vi "mmW ZMQ Handle incomming messages.vi"(11 "module loopdata":T1) -> (0 "error out":errorcluster, 3 "OK":bool)   [LabVIEW 2019, in "Communication Interface.lvlib"]
doc: "ZMQ REP:\nRecieves messages from API as ZMQ REP Socket\nParses message content into commands and triggers command user event\nWaits for command response and forwards that response back to API\nvia ZMQ"
uses:
  Communication Interface.lvlib
  module data.ctl
  Intertarget communication/CR_master_class/CR_master.lvclass
  Intertarget communication/CR slave_class/CR slave.lvclass
  ZMQ_mmWave_class/ZMQ_mmWave.lvclass
  C:/Barkhausen mmWave radar/Development/modules/mmw_instrument/src_LabVIEW/Host/Intertarget communication/CR slave_class/CR slave.lvclass
  mmw_command_lib/src_LabVIEW/mmW_commands/TypeDefs/commands.ctl
  mmw_command_lib/src_LabVIEW/mmW_commands/replies/reply_statuscode.ctl
  Intertarget communication/Error response.ctl
  mmw_command_lib/src_LabVIEW/mmW_commands/commands/typedefs/mode.ctl
  SubVIs/Shared/CMD Configure RF.ctl
  SubVIs/Shared/CMD SetFS.ctl
  SubVIs/Shared/CMD Enable.ctl
  <vilib>/event_ctls.llb/usereventprio.ctl
  SubVIs/Shared/CMD Start.ctl
  mmw_command_lib/src_LabVIEW/mmW_commands/commands/typedefs/datatypes_.ctl
  SubVIs/Shared/CMD Trigger burst.ctl
  SubVIs/mmWave instrument_class/BurstMode.ctl
  SubVIs/IQBurst_memo_class/IQBurst_memo.lvclass
  C:/Barkhausen mmWave radar/Development/modules/mmw_instrument/src_LabVIEW/Host/SubVIs/mmWave data_class/mmWave data.lvclass
  mmw_command_lib/src_LabVIEW/mmW_commands/commands/typedefs/burst_mode.ctl
  mmw_command_lib/src_LabVIEW/mmW_commands/TypeDefs/response status.ctl
  SubVIs/Shared/Config state.ctl
  SubVIs/mmWave instrument_class/System info.ctl
  SubVIs/mmWave instrument_class/System state.ctl
  SubVIs/mmWave instrument_class/Instrument state.ctl
  SubVIs/mmWave instrument_class/Instrument mode.ctl
  SubVIs/mmWave instrument_class/Sync mode.ctl
  SubVIs/mmWave instrument_class/RF port info.ctl
  4d978cd8-de24-491d-9e02-cf2f9c928746.vi
  97d28283-8354-4fd1-aa63-0fed811ffe26.vi
  <vilib>/Utility/High Resolution Relative Seconds.vi
  <vilib>/Utility/error.llb/Clear Errors.vi
  SubVIs/Shared/Comm GV.vi
  SubVIs/Shared/System GV.vi
  Log/Log GV.vi
  SubVIs/Shared/Shared.lvlib
  mmw_command_lib/src_LabVIEW/mmW_commands/mmW_commands.lvlib
  <vilib>/addons/_JKI.lib/Serialization/JSON/JKI JSON Serialization.lvlib
  SubVIs/mmWave instrument_class/mmWave instrument.lvclass
  Intertarget communication/CommandResponse communication.lvlib
  Log/Log.lvlib
panel:
  out "fs (Hz)":dbl=3072000000.0
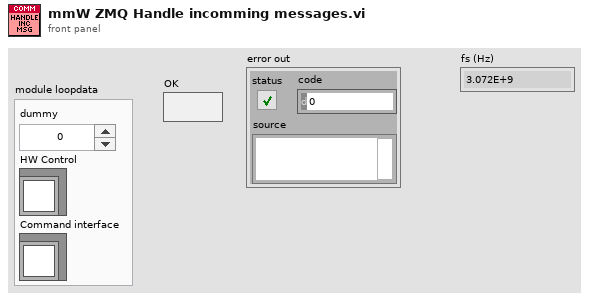
[diagram p1: front panel]
types:
  T1 = typedef "Communication Interface.lvlib/module data.ctl" = cluster{"dummy":dbl, "HW Control":refnum<class "CR_master.lvclass">, "Command interface":refnum<class "CR slave.lvclass">}
  T2 = typedef "mmW_commands.lvlib/commands.ctl" = enum16{"configure_fs", "configure_rf", "configure_trigger", "equalization_enable", "equalization_start", "lo_sync_enable", "equalization_stop", "get_instrument_status", "get_versions", "initialize_hw", "pop_rx", "set_log_level", "Shutdown", "start", "start_instrument_app", "stop", "trans", "transceive", "trigger_burst", "trigger_sync_enable", "Write TX", "resp_generic", "resp_waveform", "send_trigger", "fetch", "transceive2"}
  T3 = typedef "mmW_commands.lvlib/reply_statuscode.ctl" = enum16{"Error", "OK"}
  T4 = typedef "mmW_commands.lvlib/datatypes_.ctl" = enum16{"none", "string", "interleaved_I16", "interleaved_I32", "I16_array", "I32_array", "JSONstring"}
  T5 = typedef "mmW_commands.lvlib/response status.ctl" = enum16{"OK", "Error", "Warning", "Unknown"}
  T6 = typedef "CommandResponse communication.lvlib/Error response.ctl" = cluster{"code":i32, "message":string, "source":string}
  T7 = typedef "mmW_commands.lvlib/mode.ctl" = enum16{"RF", "IF", "BB"}
  T8 = typedef "Shared.lvlib/CMD Configure RF.ctl" = cluster{"port":string, "fc":dbl, "gain":dbl}
  T9 = typedef "Shared.lvlib/CMD SetFS.ctl" = cluster{"port":string, "fs":dbl}
  T10 = typedef "Shared.lvlib/CMD Enable.ctl" = cluster{"Enable":bool}
  T11 = typedef "usereventprio.ctl" = enum32{"high priority", "normal priority"}
  T12 = typedef "Shared.lvlib/CMD Start.ctl" = cluster{"Bursts":string[], "Acquisition duration":dbl}
  T13 = typedef "Shared.lvlib/CMD Trigger burst.ctl" = cluster{"Burst name":string, "Burst mode":T14}
  T14 = typedef "mmWave instrument.lvclass/BurstMode.ctl" = enum16{"burst", "continuous"}
  T15 = typedef "mmW_commands.lvlib/ports.ctl" = enum16{"rx", "tx"}
  T16 = cluster{"Boolean Round":bool, "code":i32, "source":string}
  T17 = typedef "mmW_commands.lvlib/burst_mode.ctl" = enum16{"burst", "continuous"}
  T18 = typedef "Shared.lvlib/Config state.ctl" = cluster{"system info":T19, "state":T20, "tx":T24, "rx":T24, "versions":cluster{"app":string, "tx fpga":string, "rx fpga":string}}
  T19 = typedef "mmWave instrument.lvclass/System info.ctl" = cluster{"mmw instr":string, "max fs":dbl, "RX/LO1 src":string, "TX/LO1 src":string, "LO2 src":string, "RX LO1 export":bool, "TX LO1 export":bool, "LO2 export":bool, "TX LO1 export level":dbl, "RX LO1 export level":dbl, "LO2 export level":dbl}
  T20 = typedef "mmWave instrument.lvclass/System state.ctl" = cluster{"hw state":T21, "lo sync en":bool, "trig sync en":bool, "mode":T22, "sync":T23, "equalization en":bool}
  T21 = typedef "mmWave instrument.lvclass/Instrument state.ctl" = enum16{"Off", "Initialization", "Configuration", "Running", "Calibration"}
  T22 = typedef "mmWave instrument.lvclass/Instrument mode.ctl" = enum16{"RF", "IF", "BB"}
  T23 = typedef "mmWave instrument.lvclass/Sync mode.ctl" = enum16{"Slave", "Master"}
  T24 = typedef "mmWave instrument.lvclass/RF port info.ctl" = cluster{"fc":dbl, "gain":dbl, "fs":dbl, "trigger delay":dbl}
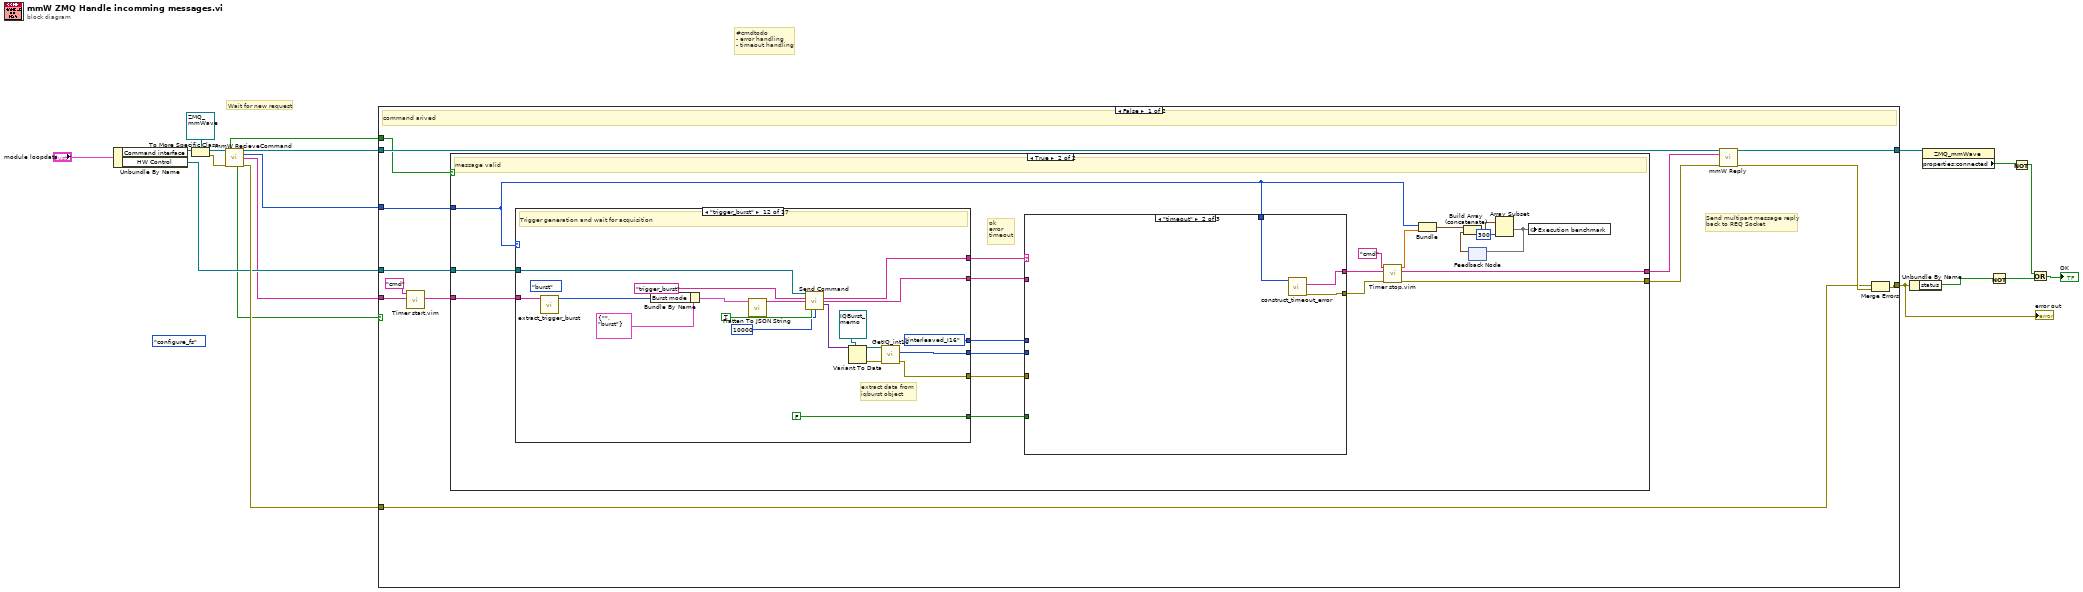
[diagram p0: block diagram]
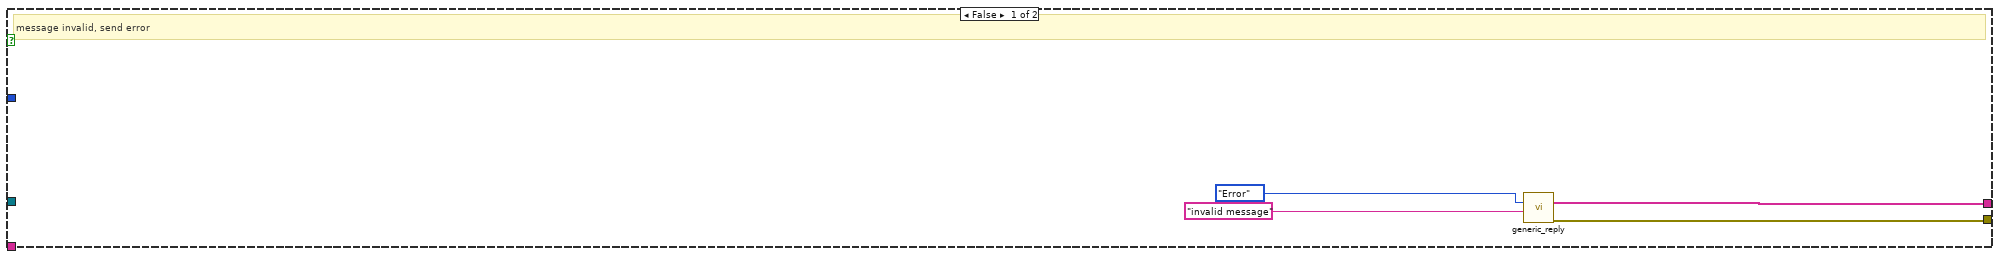
[diagram p2: hidden frame]
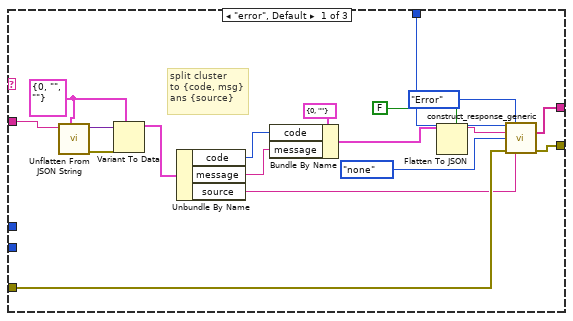
[diagram p3: hidden frame]
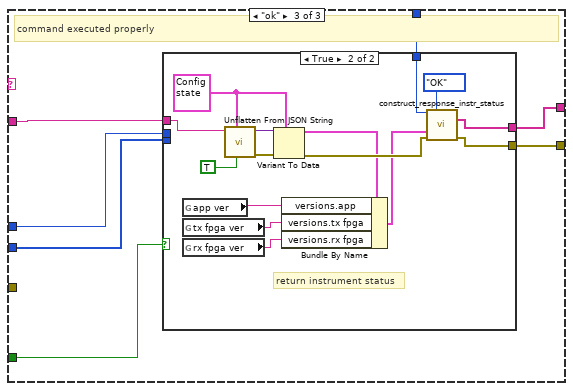
[diagram p4: hidden frame]
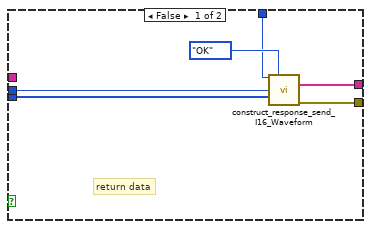
[diagram p5: hidden frame]
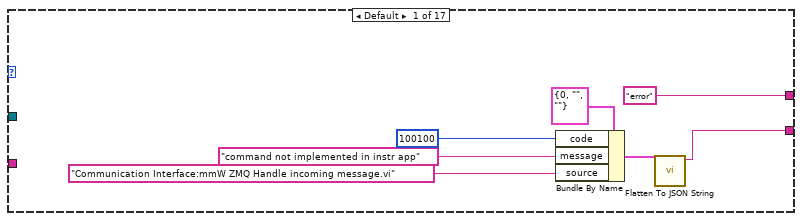
[diagram p6: hidden frame]
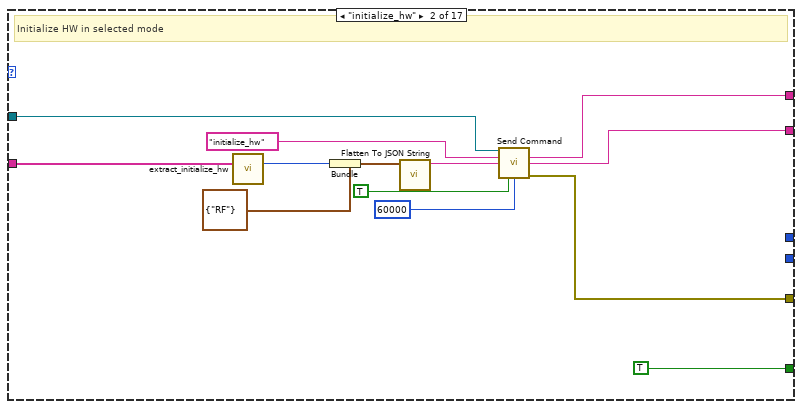
[diagram p7: hidden frame]
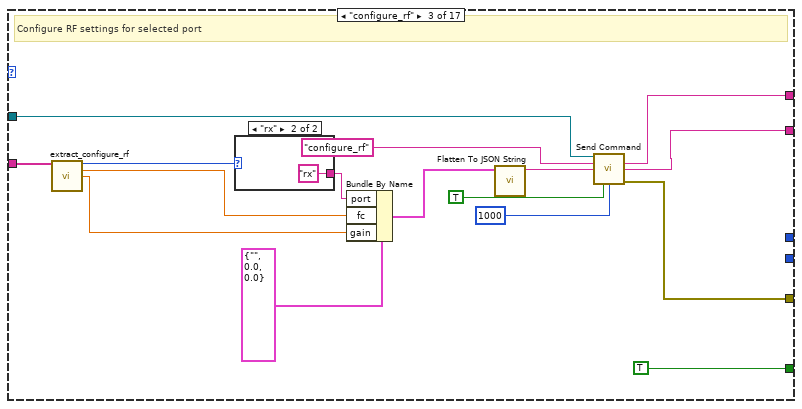
[diagram p8: hidden frame]
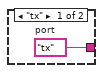
[diagram p9: hidden frame]
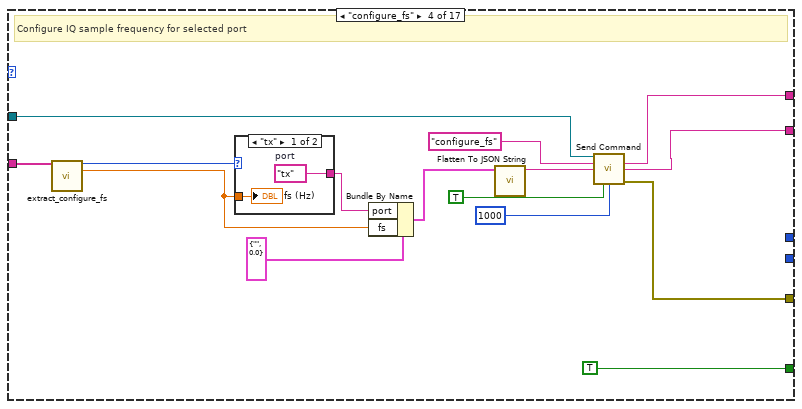
[diagram p10: hidden frame]
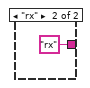
[diagram p11: hidden frame]
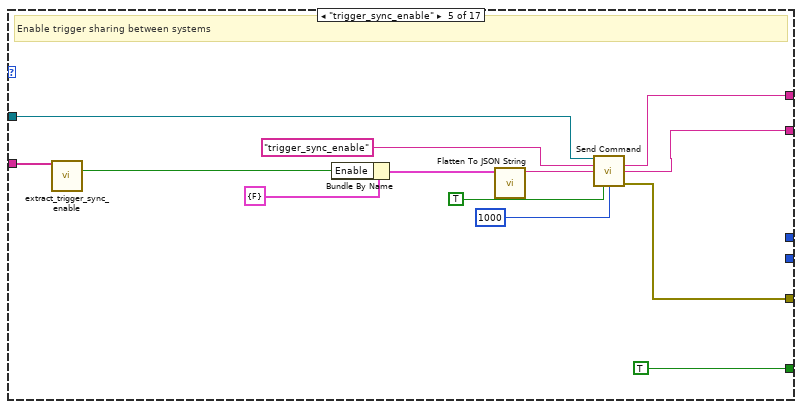
[diagram p12: hidden frame]
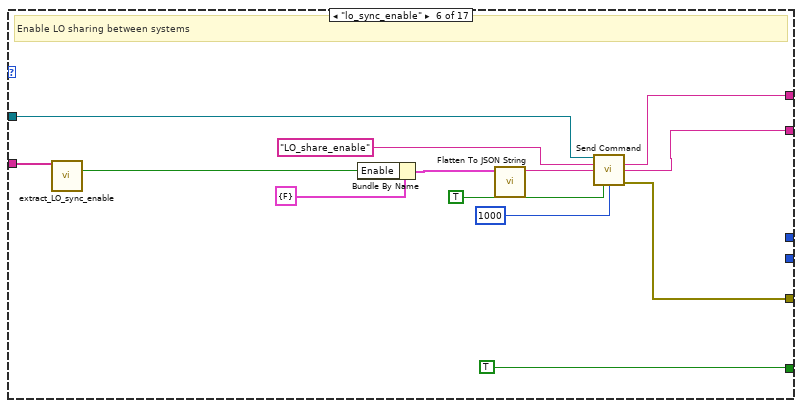
[diagram p13: hidden frame]
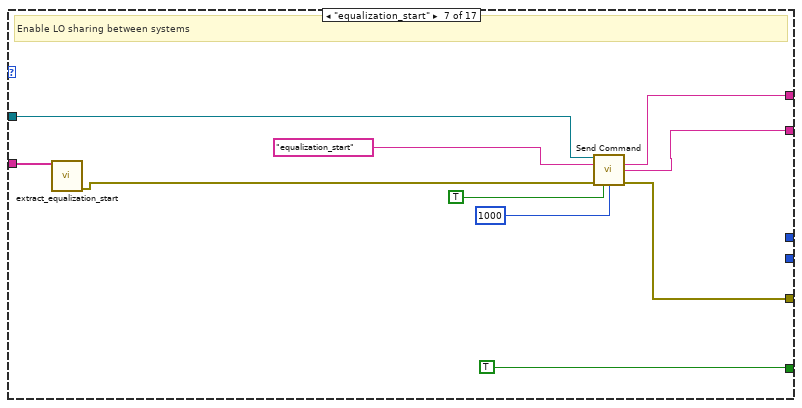
[diagram p14: hidden frame]
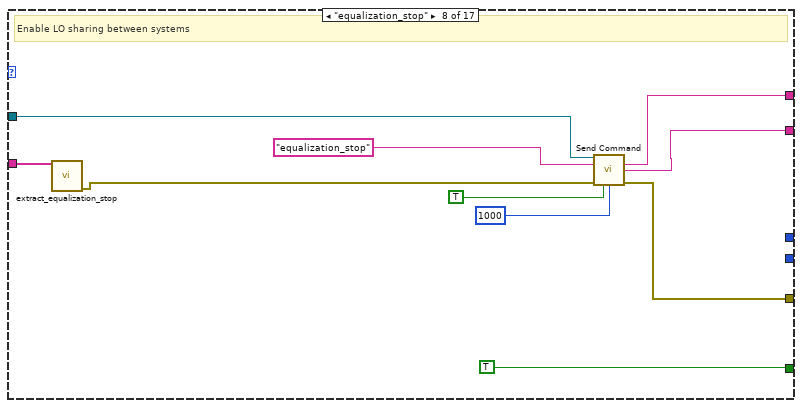
[diagram p15: hidden frame]
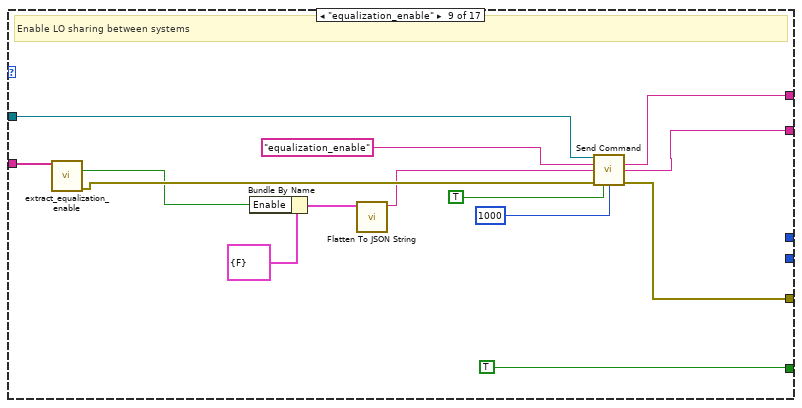
[diagram p16: hidden frame]
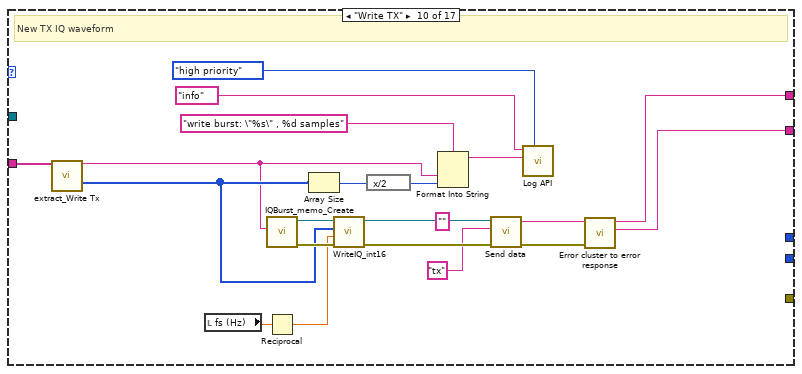
[diagram p17: hidden frame]
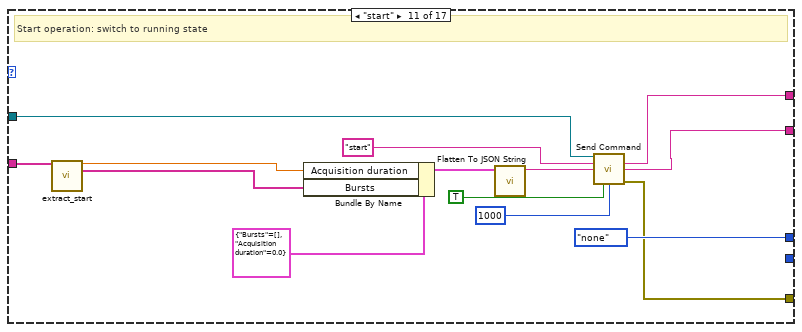
[diagram p18: hidden frame]
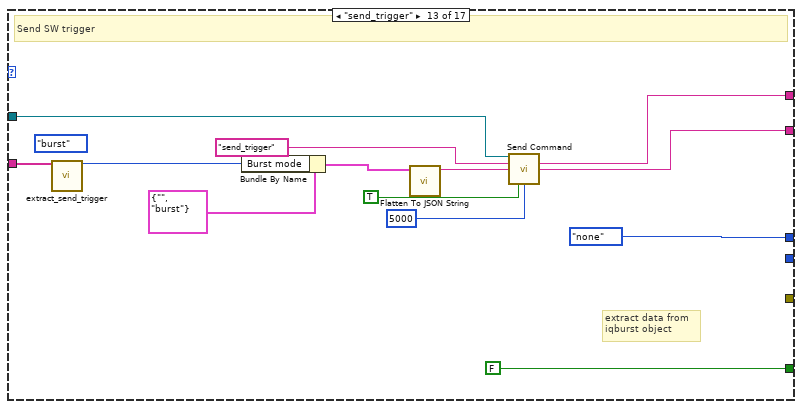
[diagram p19: hidden frame]
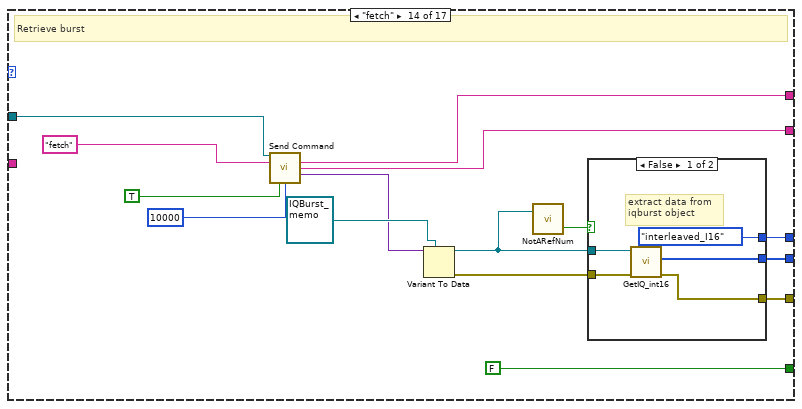
[diagram p20: hidden frame]
diagram:
  (unwired) commands."configure_fs" ("command out")
  # "Wait for new request"
  # "#cmdtodo\n- error handling\n- timeout handling"
  n1 = Unbundle By Name("module loopdata") -> ("Command interface"=w10:refnum<class "CR slave.lvclass">, "HW Control"=w11:refnum<class "CR_master.lvclass">)
  n2 = To More Specific Class(target class=refnum<class "ZMQ_mmWave.lvclass"> refnum ("CommandResponse communication.lvlib:ZMQ_mmWave"), reference=w10) -> (specific class reference=w8:refnum<class "ZMQ_mmWave.lvclass">, error out=w3:errorcluster)  [unwired: 1 in]
  n3 = call-dynamic "mmW RecieveCommand.vi"("reference in"=w8, "error in (no error)"=w3) -> ("Valid message?"=w2:bool, "reference out"=w12:refnum<class "ZMQ_mmWave.lvclass">, "command out"=w5:T2, "multipart message"=w4:string[], "timed out?"=w6:bool, "error out"=w13:errorcluster)  [unwired: 8 in]
  n4 = case shown="False" w6 {
    tunnel: w11 -> [w32 _]
    tunnel: w12 -> [w31 w359]
    tunnel: w13 -> [w27 w360]
    tunnel: [w28 w360] -> w14
    tunnel: [w30 w359] -> w15
    tunnel: w5 -> [w26 _]
    tunnel: w4 -> [w22 _]
    tunnel: w2 -> [w25 _]
    frame False {
      # "Send multipart message reply\nback to REQ Socket"
      # "command arived"
      n5 = call "Timer start.vim"("dataflow in"=w22, "timer in (t1)"="cmd" ("timer name (t1)")) -> ("dataflow out"=w21:string[])  [unwired: 8 in, 1 out]
      n6 = case shown="True" w25 {
        tunnel: w32 -> [_ w55]
        tunnel: w26 -> [_ w44]
        tunnel: w21 -> [_ w54]
        tunnel: [w36 w45] -> w24
        tunnel: [w33 w50] -> w23
        frame False {
          # "message invalid, send error"
          n7 = call "generic_reply.vi"("Status (Error)"=reply_statuscode."Error", "(error code)"="invalid message" ("Response out")) -> ("multipart message"=w36:string[], "error out"=w33:errorcluster)  [unwired: 11 in, 1 out]
        }
        frame True {
          # "ok\nerror\ntimeout"
          # "message valid"
          n8 = case shown="\"trigger_burst\"" w44 {
            tunnel: w55 -> [_ w114 w135 w152 w168 w181 w192 w202 w216 _ w249 w268 w281 w287 w313 w348 _]
            tunnel: w54 -> [_ w122 w140 w157 w173 w186 w196 w206 w220 w231 w254 w273 w286 _ w317 w347 _]
            tunnel: ["error" ("status") w116 w129 w147 w166 w179 w191 w201 w215 w234 w246 w255 w274 w288 w310 w346 _] -> w53
            tunnel: [w105 w115 w128 w146 w165 w178 w190 w200 w214 w233 w245 w265 w278 w298 w312 w345 _] -> w52
            tunnel: [_ _ _ _ _ _ _ _ _ _ _ w259 _ w294 _ w343 _] -> w51
            tunnel: [_ _ _ _ _ _ _ _ _ _ datatypes_."none" ("datatype") datatypes_."interleaved_I16" ("datatype") datatypes_."none" ("datatype") w293 _ w344 _] -> w49
            tunnel: [_ w113 w126 w145 w164 w177 w189 w199 w213 _ w241 w257 _ w292 w311 w326 _] -> w48
            tunnel: [_ TRUE TRUE TRUE TRUE TRUE TRUE TRUE TRUE _ _ FALSE FALSE FALSE _ _ _] -> w42
            frame Default {
              n9 = Bundle By Name(cluster=T6 {"code"=0, "message"="", "source"=""} ("Error response"), "code"=100100, "message"="command not implemented in instr app", "source"="Communication Interface:mmW ZMQ Handle incoming message.vi" ("message")) -> (w106:T6)
              n10 = call <vilib>:"Flatten To JSON String.vi"("Variant"=w106) -> ("JSON String"=w105:string)  [unwired: 9 in, 1 out]
            }
            frame "initialize_hw" {
              # "Initialize HW in selected mode"
              n11 = call "extract_initialize_hw.vi"("multipart message in"=w122) -> ("Mode"=w120:T7)  [unwired: 10 in, 4 out]
              n12 = Bundle(cluster=cluster{"mode":T7} {"mode"=enum."RF"}, "mode"=w120) -> (w118:cluster{"mode":T7})
              n13 = call <vilib>:"Flatten To JSON String.vi"("Variant"=w118) -> ("JSON String"=w119:string)  [unwired: 9 in, 1 out]
              n14 = call-dynamic "Send Command.vi"("reference in"=w114, "message"="initialize_hw", "parameters"=w119, "response?"=TRUE, "timeout"=60000) -> ("status"=w116:string, "reponse"=w115:string, "error out"=w113:errorcluster)  [unwired: 6 in, 2 out]
            }
            frame "configure_rf" {
              # "Configure RF settings for selected port"
              n15 = call "extract_configure_rf.vi"("multipart message in"=w140) -> ("ports"=w133:T15, "fc (Hz)"=w132:dbl, "gain"=w127:dbl)  [unwired: 9 in, 3 out]
              n16 = case shown="\"rx\"" w133 {
                tunnel: [w141 "rx" ("port")] -> w131
                frame "tx" {
                  w141 = "tx"  # port
                }
                frame "rx" {
                }
              }
              n17 = Bundle By Name(cluster=T8 {"port"="", "fc"=0.0, "gain"=0.0}, "port"=w131, "fc"=w132, "gain"=w127) -> (w130:T8)
              n18 = call <vilib>:"Flatten To JSON String.vi"("Variant"=w130) -> ("JSON String"=w136:string)  [unwired: 9 in, 1 out]
              n19 = call-dynamic "Send Command.vi"("reference in"=w135, "message"="configure_rf", "parameters"=w136, "response?"=TRUE, "timeout"=1000) -> ("status"=w129:string, "reponse"=w128:string, "error out"=w126:errorcluster)  [unwired: 6 in, 2 out]
            }
            frame "configure_fs" {
              # "Configure IQ sample frequency for selected port"
              n20 = call "extract_configure_fs.vi"("multipart message in"=w157) -> ("ports"=w150:T15, "fs (Hz)"=w143:dbl)  [unwired: 10 in, 3 out]
              n21 = case shown="\"tx\"" w150 {
                tunnel: [w159 "rx" ("port")] -> w149
                tunnel: w143 -> [w158 _]
                frame "tx" {
                  w159 = "tx"  # port
                  "fs (Hz)" <- w158
                }
                frame "rx" {
                }
              }
              n22 = Bundle By Name(cluster=T9 {"port"="", "fs"=0.0}, "port"=w149, "fs"=w143) -> (w148:T9)
              n23 = call <vilib>:"Flatten To JSON String.vi"("Variant"=w148) -> ("JSON String"=w153:string)  [unwired: 9 in, 1 out]
              n24 = call-dynamic "Send Command.vi"("reference in"=w152, "message"="configure_fs", "parameters"=w153, "response?"=TRUE, "timeout"=1000) -> ("status"=w147:string, "reponse"=w146:string, "error out"=w145:errorcluster)  [unwired: 6 in, 2 out]
            }
            frame "trigger_sync_enable" {
              # "Enable trigger sharing between systems"
              n25 = call "extract_trigger_sync_enable.vi"("multipart message in"=w173) -> ("Enable"=w162:bool)  [unwired: 11 in, 3 out]
              n26 = Bundle By Name(cluster=T10 {"Enable"=FALSE} ("Equalization command"), "Enable"=w162) -> (w167:T10)
              n27 = call <vilib>:"Flatten To JSON String.vi"("Variant"=w167) -> ("JSON String"=w169:string)  [unwired: 9 in, 1 out]
              n28 = call-dynamic "Send Command.vi"("reference in"=w168, "message"="trigger_sync_enable", "parameters"=w169, "response?"=TRUE, "timeout"=1000) -> ("status"=w166:string, "reponse"=w165:string, "error out"=w164:errorcluster)  [unwired: 6 in, 2 out]
            }
            frame "lo_sync_enable" {
              # "Enable LO sharing between systems"
              n29 = call "extract_LO_sync_enable.vi"("multipart message in"=w186) -> ("Enable"=w175:bool)  [unwired: 11 in, 3 out]
              n30 = Bundle By Name(cluster=T10 {"Enable"=FALSE} ("Equalization command"), "Enable"=w175) -> (w180:T10)
              n31 = call <vilib>:"Flatten To JSON String.vi"("Variant"=w180) -> ("JSON String"=w182:string)  [unwired: 9 in, 1 out]
              n32 = call-dynamic "Send Command.vi"("reference in"=w181, "message"="LO_share_enable", "parameters"=w182, "response?"=TRUE, "timeout"=1000) -> ("status"=w179:string, "reponse"=w178:string, "error out"=w177:errorcluster)  [unwired: 6 in, 2 out]
            }
            frame "equalization_start" {
              # "Enable LO sharing between systems"
              n33 = call "extract_equalization_start.vi"("multipart message in"=w196) -> ("error out"=w187:errorcluster)  [unwired: 12 in, 2 out]
              n34 = call-dynamic "Send Command.vi"("reference in"=w192, "message"="equalization_start", "error in (no error)"=w187, "response?"=TRUE, "timeout"=1000) -> ("status"=w191:string, "reponse"=w190:string, "error out"=w189:errorcluster)  [unwired: 6 in, 2 out]
            }
            frame "equalization_stop" {
              # "Enable LO sharing between systems"
              n35 = call "extract_equalization_stop.vi"("multipart message in"=w206) -> ("error out"=w197:errorcluster)  [unwired: 12 in, 2 out]
              n36 = call-dynamic "Send Command.vi"("reference in"=w202, "message"="equalization_stop", "error in (no error)"=w197, "response?"=TRUE, "timeout"=1000) -> ("status"=w201:string, "reponse"=w200:string, "error out"=w199:errorcluster)  [unwired: 6 in, 2 out]
            }
            frame "equalization_enable" {
              # "Enable LO sharing between systems"
              n37 = call "extract_equalization_enable.vi"("multipart message in"=w220) -> ("Enable"=w208:bool, "error out"=w211:errorcluster)  [unwired: 11 in, 2 out]
              n38 = Bundle By Name(cluster=T10 {"Enable"=FALSE} ("Equalization command"), "Enable"=w208) -> (w209:T10)
              n39 = call <vilib>:"Flatten To JSON String.vi"("Variant"=w209) -> ("JSON String"=w207:string)  [unwired: 9 in, 1 out]
              n40 = call-dynamic "Send Command.vi"("reference in"=w216, "message"="equalization_enable", "parameters"=w207, "error in (no error)"=w211, "response?"=TRUE, "timeout"=1000) -> ("status"=w215:string, "reponse"=w214:string, "error out"=w213:errorcluster)  [unwired: 5 in, 2 out]
            }
            frame "Write TX" {
              # "New TX IQ waveform"
              n41 = call "extract_Write Tx.vi"("multipart message in"=w231) -> ("burstname"=w224:string, "interleaved I16 wfm"=w228:i16[])  [unwired: 9 in, 4 out]
              n42 = local read "fs (Hz)"() -> (w222:dbl)
              n43 = call "IQBurst_memo_Create.vi"("burst name"=w224) -> ("error out"=w239:errorcluster, "reference out"=w240:refnum<class "IQBurst_memo.lvclass">)  [unwired: 9 in]
              n44 = Reciprocal(x=w222) -> (1/x=w221:dbl)
              n45 = Array Size(array=w228) -> (size(s)=w227:i32)
              n46 = call-dynamic "WriteIQ_int16.vi"("error in (no error)"=w239, "dt"=w221, "data"=w228, "reference in"=w240) -> ("error out"=w237:errorcluster, "reference out"=w238:refnum<class "IQBurst_memo.lvclass">)  [unwired: 6 in]
              n47 = expression code="x/2"(w227) -> (w225:i32)
              n48 = Format Into String(format string="write burst: \"%s\" , %d samples", w224, w225) -> (resulting string=w223:string)  [unwired: 2 in, 1 out]
              n49 = call "Send data.vi"("error in (no error)"=w237, "group"="tx", "Data"=w238) -> ("error out"=w236:T16)  [unwired: 8 in]
              n50 = call "Log API.vi"("priority (normal)"=usereventprio."high priority", "data"=w223, "message"="info") -> ()  [unwired: 8 in, 1 out]
              n51 = call "Error cluster to error response.vi"("error in (no error)"=w236, "response"="" ("message")) -> ("JSON String"=w233:string, "message"=w234:string)  [unwired: 8 in]
            }
            frame "start" {
              # "Start operation: switch to running state"
              n52 = call "extract_start.vi"("multipart message in"=w254) -> ("acq_length (ms)"=w244:dbl, "bursts"=w243:string[])  [unwired: 10 in, 3 out]
              n53 = Bundle By Name(cluster=T12 {"Bursts"=[], "Acquisition duration"=0.0}, "Acquisition duration"=w244, "Bursts"=w243) -> (w247:T12)
              n54 = call <vilib>:"Flatten To JSON String.vi"("Variant"=w247) -> ("JSON String"=w250:string)  [unwired: 9 in, 1 out]
              n55 = call-dynamic "Send Command.vi"("reference in"=w249, "message"="start", "parameters"=w250, "response?"=TRUE, "timeout"=1000) -> ("status"=w246:string, "reponse"=w245:string, "error out"=w241:errorcluster)  [unwired: 6 in, 2 out]
            }
            frame "trigger_burst" {
              (unwired) burst_mode."burst" ("burst_mode")
              # "extract data from \niqburst object"
              # "Trigger generation and wait for acquisition"
              n56 = call "extract_trigger_burst.vi"("multipart message in"=w273) -> ("burst_mode"=w264:T17)  [unwired: 10 in, 4 out]
              n57 = Bundle By Name(cluster=T13 {"Burst name"="", "Burst mode"=enum."burst"}, "Burst mode"=w264) -> (w266:T13)
              n58 = call <vilib>:"Flatten To JSON String.vi"("Variant"=w266) -> ("JSON String"=w269:string)  [unwired: 9 in, 1 out]
              n59 = call-dynamic "Send Command.vi"("reference in"=w268, "message"="trigger_burst", "parameters"=w269, "response?"=TRUE, "timeout"=10000) -> ("status"=w255:string, "reponse"=w265:string, "data"=w260:variant)  [unwired: 6 in, 2 out]
              n60 = Variant To Data(type=refnum<class "IQBurst_memo.lvclass"> refnum ("reference out"), Variant=w260) -> (data=w262:refnum<class "IQBurst_memo.lvclass">, error out=w261:errorcluster)  [unwired: 1 in]
              n61 = call-dynamic "GetIQ_int16.vi"("error in (no error)"=w261, "reference in"=w262) -> ("error out"=w257:errorcluster, "data"=w259:i16[])  [unwired: 6 in, 2 out]
            }
            frame "send_trigger" {
              (unwired) burst_mode."burst" ("burst_mode")
              # "extract data from \niqburst object"
              # "Send SW trigger"
              n62 = call "extract_send_trigger.vi"("multipart message in"=w286) -> ("burst_mode"=w277:T17)  [unwired: 11 in, 3 out]
              n63 = Bundle By Name(cluster=T13 {"Burst name"="", "Burst mode"=enum."burst"}, "Burst mode"=w277) -> (w279:T13)
              n64 = call <vilib>:"Flatten To JSON String.vi"("Variant"=w279) -> ("JSON String"=w282:string)  [unwired: 9 in, 1 out]
              n65 = call-dynamic "Send Command.vi"("reference in"=w281, "message"="send_trigger", "parameters"=w282, "response?"=TRUE, "timeout"=5000) -> ("status"=w274:string, "reponse"=w278:string)  [unwired: 6 in, 3 out]
            }
            frame "fetch" {
              # "Retrieve burst"
              n66 = call-dynamic "Send Command.vi"("reference in"=w287, "message"="fetch", "response?"=TRUE, "timeout"=10000) -> ("status"=w288:string, "reponse"=w298:string, "data"=w295:variant)  [unwired: 7 in, 2 out]
              n67 = Variant To Data(type=refnum<class "IQBurst_memo.lvclass"> refnum ("reference out"), Variant=w295) -> (data=w290:refnum<class "IQBurst_memo.lvclass">, error out=w296:errorcluster)  [unwired: 1 in]
              n68 = call-dynamic "NotARefNum.vi"("reference in"=w290) -> ("not a refnum?"=w289:bool)  [unwired: 1 in, 1 out]
              n69 = case shown="False" w289 {
                tunnel: w296 -> [w306 _]
                tunnel: [w305 i16[] [] ("data")] -> w294
                tunnel: [datatypes_."interleaved_I16" ("datatype") datatypes_."none" ("datatype")] -> w293
                tunnel: [w303 errorcluster {"status"=FALSE, "code"=0, "source"=""} ("error out")] -> w292
                tunnel: w290 -> [w302 _]
                frame False {
                  # "extract data from \niqburst object"
                  n70 = call-dynamic "GetIQ_int16.vi"("error in (no error)"=w306, "reference in"=w302) -> ("error out"=w303:errorcluster, "data"=w305:i16[])  [unwired: 6 in, 2 out]
                }
                frame True {
                  # "empty data"
                }
              }
            }
            frame "stop" {
              # "Stop operation"
              n71 = call "extract_stop.vi"("multipart message in"=w317) -> ()  [unwired: 12 in, 3 out]
              n72 = call-dynamic "Send Command.vi"("reference in"=w313, "message"="stop", "response?"=TRUE, "timeout"=1000) -> ("status"=w310:string, "reponse"=w312:string, "error out"=w311:errorcluster)  [unwired: 7 in, 2 out]
            }
            frame "transceive" {
              n73 = call "extract_transceive.vi"("multipart message in"=w347) -> ("acq_length"=w327:dbl, "burstname"=w320:string, "bursts"=w321:string[], "Interleaved I16 wfm"=w336:i16[])  [unwired: 7 in, 4 out]
              n74 = feedback #1(0) -> (w325:i32)
              n75 = Increment(x=w325) -> (x+1=w323:i32)
              n76 = feedback-in #1(w323) -> ()
              n77 = Number To Decimal String(number=w323) -> (decimal integer string=w322:string)  [unwired: 1 in]
              n78 = Bundle By Name(cluster=T12 {"Bursts"=[], "Acquisition duration"=0.0} ("Start command"), "Acquisition duration"=w327, "Bursts"=w321) -> (w329:T12)
              n79 = Build Array(w322) -> ()  [unwired: 1 out]
              n80 = local read "fs (Hz)"() -> (w319:dbl)
              n81 = call "IQBurst_memo_Create.vi"("burst name"=w320) -> ("error out"=w339:errorcluster, "reference out"=w340:refnum<class "IQBurst_memo.lvclass">)  [unwired: 9 in]
              n82 = Reciprocal(x=w319) -> (1/x=w318:dbl)
              n83 = call <vilib>:"Flatten To JSON String.vi"("Variant"=w329) -> ("JSON String"=w328:string)  [unwired: 9 in, 1 out]
              n84 = call-dynamic "WriteIQ_int16.vi"("error in (no error)"=w339, "dt"=w318, "data"=w336, "reference in"=w340) -> ("reference out"=w338:refnum<class "IQBurst_memo.lvclass">)  [unwired: 6 in, 1 out]
              n85 = call-dynamic "Send Command.vi"("reference in"=w348, "message"="transcieve", "parameters"=w328, "data"=w338, "response?"=TRUE, "timeout"=60000) -> ("status"=w346:string, "reponse"=w345:string, "data"=w331:variant)  [unwired: 5 in, 2 out]
              n86 = Variant To Data(type=refnum<class "IQBurst_memo.lvclass"> refnum ("reference out"), Variant=w331) -> (data=w333:refnum<class "IQBurst_memo.lvclass">, error out=w334:errorcluster)  [unwired: 1 in]
              n87 = call-dynamic "NotARefNum.vi"("reference in"=w333) -> ("not a refnum?"=w332:bool)  [unwired: 1 in, 1 out]
              n88 = case shown="False" w332 {
                tunnel: w334 -> [w353 _]
                tunnel: [w352 i16[] [] ("data")] -> w343
                tunnel: [datatypes_."interleaved_I16" ("datatype") datatypes_."none" ("datatype")] -> w344
                tunnel: [w350 errorcluster {"status"=FALSE, "code"=0, "source"=""} ("error out")] -> w326
                tunnel: w333 -> [w349 _]
                frame False {
                  # "extract data from \niqburst object"
                  n89 = call-dynamic "GetIQ_int16.vi"("error in (no error)"=w353, "reference in"=w349) -> ("error out"=w350:errorcluster, "data"=w352:i16[])  [unwired: 6 in, 2 out]
                }
                frame True {
                  # "empty data"
                }
              }
            }
            frame "Shutdown" {
              # "Close application"
              n90 = global read "Comm GV.vi" "CloseApp"() -> (w358:refnum<user-event>)
              n91 = Generate User Event(user event=w358, event data cluster=TRUE ("event data")) -> ()  [unwired: 2 in, 2 out]
            }
          }
          n92 = case shown="\"timeout\"" w53 {
            tunnel: w44 -> [w73 w76 w79]
            tunnel: w52 -> [w67 _ w77]
            tunnel: w51 -> [_ _ w83]
            tunnel: [w70 w75 w82] -> w46
            tunnel: [w69 w74 w81] -> w50
            tunnel: w49 -> [_ _ w80]
            tunnel: w48 -> [w68 _ _]
            tunnel: w42 -> [_ _ w78]
            frame "error", Default {
              w64 = T6 {"code"=0, "message"="", "source"=""} ("Error response")
              # "split cluster\nto {code, msg}\nans {source}"
              n93 = call <vilib>:"Unflatten From JSON String.vi"("Type and Defaults"=w64, "JSON String"=w67) -> ("error out"=w66:errorcluster, "Variant"=w65:variant)  [unwired: 8 in]
              n94 = Variant To Data(error in=w66, type=w64, Variant=w65) -> (data=w63:T6)  [unwired: 1 out]
              n95 = Unbundle By Name(w63) -> ("code"=w60:i32, "message"=w59:string, "source"=w62:string)
              n96 = Bundle By Name(cluster=cluster{"code":i32, "message":string} {"code"=0, "message"=""} ("Error response"), "code"=w60, "message"=w59) -> (w58:cluster{"code":i32, "message":string})
              n97 = Flatten To JSON(enable LabVIEW extensions? (T)=FALSE, anything=w58) -> (JSON string=w57:string)  [unwired: 1 in, 1 out]
              n98 = call "construct_response_generic.vi"("command in"=w73, "Status"=response_status."Error", "generic_info"=w57, "datatype"=datatypes_."none", "error in (no error) 2"=w68, "source"=w62) -> ("Multipart message"=w70:string[], "error out 2"=w69:errorcluster)  [unwired: 6 in, 2 out]
            }
            frame "timeout" {
              n99 = call "construct_timeout_error.vi"("command in"=w76) -> ("Multipart message"=w75:string[], "error out 2"=w74:errorcluster)  [unwired: 12 in, 1 out]
            }
            frame "ok" {
              # "command executed properly"
              n100 = case shown="True" w78 {
                tunnel: w83 -> [w88 _]
                tunnel: [w87 w99] -> w82
                tunnel: [w86 w98] -> w81
                tunnel: w80 -> [w85 _]
                tunnel: w79 -> [w84 w101]
                tunnel: w77 -> [_ w102]
                frame False {
                  # "return data"
                  n101 = call "construct_response_send_I16_Waveform.vi"("command in"=w84, "Status"=response_status."OK", "datatype"=w85, "I16 waveform in"=w88) -> ("Multipart message"=w87:string[], "error out 2"=w86:errorcluster)  [unwired: 9 in, 1 out]
                }
                frame True {
                  w95 = T18 {"system info"={"mmw instr"="", "max fs"=0.0, "RX/LO1 src"="", "TX/LO1 src"="", "LO2 src"="", "RX LO1 export"=FALSE, "TX LO1 export"=FALSE, "LO2 export"=FALSE, "TX LO1 export level"=0.0, "RX LO1 export level"=0.0, "LO2 export level"=0.0}, "state"={"hw state"=enum."Off", "lo sync en"=FALSE, "trig sync en"=FALSE, "mode"=enum."RF", "sync"=enum."Slave", "equalization en"=FALSE}, "tx"={"fc"=0.0, "gain"=0.0, "fs"=0.0, "trigger delay"=0.0}, "rx"={"fc"=0.0, "gain"=0.0, "fs"=0.0, "trigger delay"=0.0}, "versions"={"app"="", "tx fpga"="", "rx fpga"=""}} ("Transciever config")
                  # "return instrument status"
                  n102 = global read "System GV.vi" "app ver"() -> (w92:string)
                  n103 = global read "System GV.vi" "tx fpga ver"() -> (w91:string)
                  n104 = global read "System GV.vi" "rx fpga ver"() -> (w90:string)
                  n105 = call <vilib>:"Unflatten From JSON String.vi"("Nulls as Defaults (F)"=TRUE, "Type and Defaults"=w95, "JSON String"=w102) -> ("error out"=w104:errorcluster, "Variant"=w103:variant)  [unwired: 7 in]
                  n106 = Variant To Data(error in=w104, type=w95, Variant=w103) -> (data=w94:T18, error out=w97:errorcluster)
                  n107 = Bundle By Name(cluster=w94, "versions.app"=w92, "versions.tx fpga"=w91, "versions.rx fpga"=w90) -> (w93:T18)
                  n108 = call "construct_response_instr_status.vi"("command in"=w101, "Status"=response_status."OK", "Config"=w93, "error in (no error) 2"=w97) -> ("Multipart message"=w99:string[], "error out 2"=w98:errorcluster)  [unwired: 9 in, 1 out]
                }
              }
            }
          }
          n109 = call "Timer stop.vim"("dataflow in"=w46, "timer name (t1)"="cmd") -> ("dataflow out"=w45:string[], "final time"=w43:dbl)  [unwired: 8 in]
          n110 = Bundle("command out"=w44, "final time"=w43) -> (w41:cluster{"command out":T2, "final time":dbl})  [unwired: 1 in]
          n111 = feedback #2() -> (w40:cluster{"command out":T2, "final time":dbl}[])  [unwired: 1 in]
          n112 = Build Array (concatenate)(w41, w40) -> (w39:cluster{"command out":T2, "final time":dbl}[])
          n113 = Array Subset(array=w39, length=300) -> (w37:cluster{"command out":T2, "final time":dbl}[])  [unwired: 1 in]
          n114 = feedback-in #2(w37) -> ()
          n115 = global write "Log GV.vi" "Execution benchmark"(w37) -> ()
        }
      }
      n116 = call-dynamic "mmW Reply.vi"("reference in"=w31, "Multipart message"=w24, "error in (no error)"=w23) -> ("reference out"=w30:refnum<class "ZMQ_mmWave.lvclass">, "error out"=w29:errorcluster)  [unwired: 11 in]
      n117 = Merge Errors(w27, w29) -> (w28:errorcluster)
    }
    frame True {
      # "timeout - no new command"
    }
  }
  "error out" <- w14
  n118 = Unbundle By Name(w14) -> ("status"=w17:bool)
  n119 = property class="ZMQ_mmWave"(reference=w15) -> ("properties:connected"=w16:bool)  [unwired: 1 in, 2 out]
  n120 = Not(x=w17) -> (.not. x?=w1:bool)
  n121 = Not(x=w16) -> (.not. x?=w18:bool)
  n122 = Or(x=w18, y=w1) -> (x .or. y?=→"OK":bool)
